vi "Settings Dialog.vi"(8 "error in (no error)":errorcluster, 11 "Settings in":T1) -> (0 "error out":errorcluster, 1 "Cancelled?":bool, 2 "UI Refresh Needed?":bool, 3 "Settings out":T1)   [LabVIEW 2022 SP3, in "Settings.lvlib"]
doc: "Dialog for selecting user specified settings."
uses:
  Settings.lvlib
  Settings.ctl
  Acquisition/Network Configuration.ctl
  Logging/Logging Configuration.ctl
  <vilib>/Utility/xml.llb/Write to XML File(string).vi
  Acquisition/Acquisition.lvlib
  Logging/Logging.lvlib
panel:
  in  "IP Address":string="127.0.0.1"
  in  "Port":dbl=5005.0
  in  "Log File Path":path
  in  "Cancel Button":bool
  in  "OK Button":bool
  # "Non visible portion of dialog (needed for connector pane)."
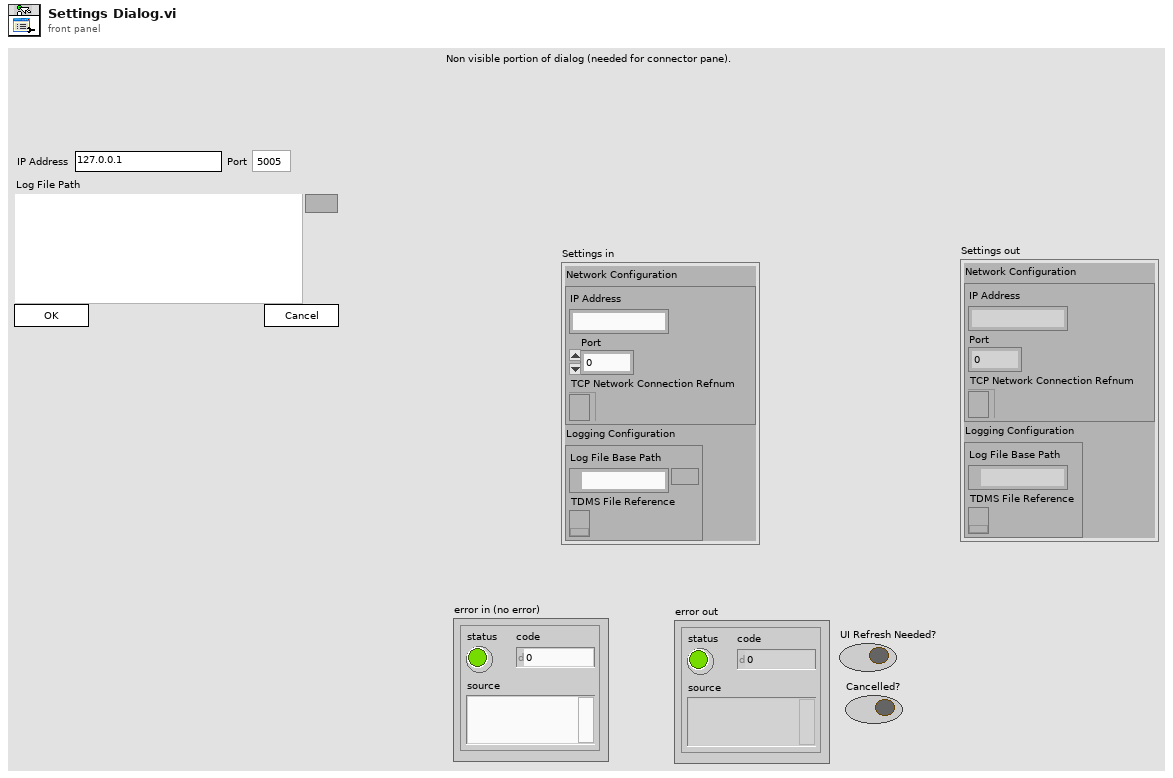
[diagram p1: front panel]
types:
  T1 = typedef "Settings.lvlib/Settings.ctl" = cluster{"Network Configuration":T2, "Logging Configuration":T3}
  T2 = typedef "Acquisition.lvlib/Network Configuration.ctl" = cluster{"IP Address":string, "Port":dbl, "TCP Network Connection Refnum":refnum<k5>}
  T3 = typedef "Logging.lvlib/Logging Configuration.ctl" = cluster{"Log File Base Path":path, "TDMS File Reference":refnum<k34>}
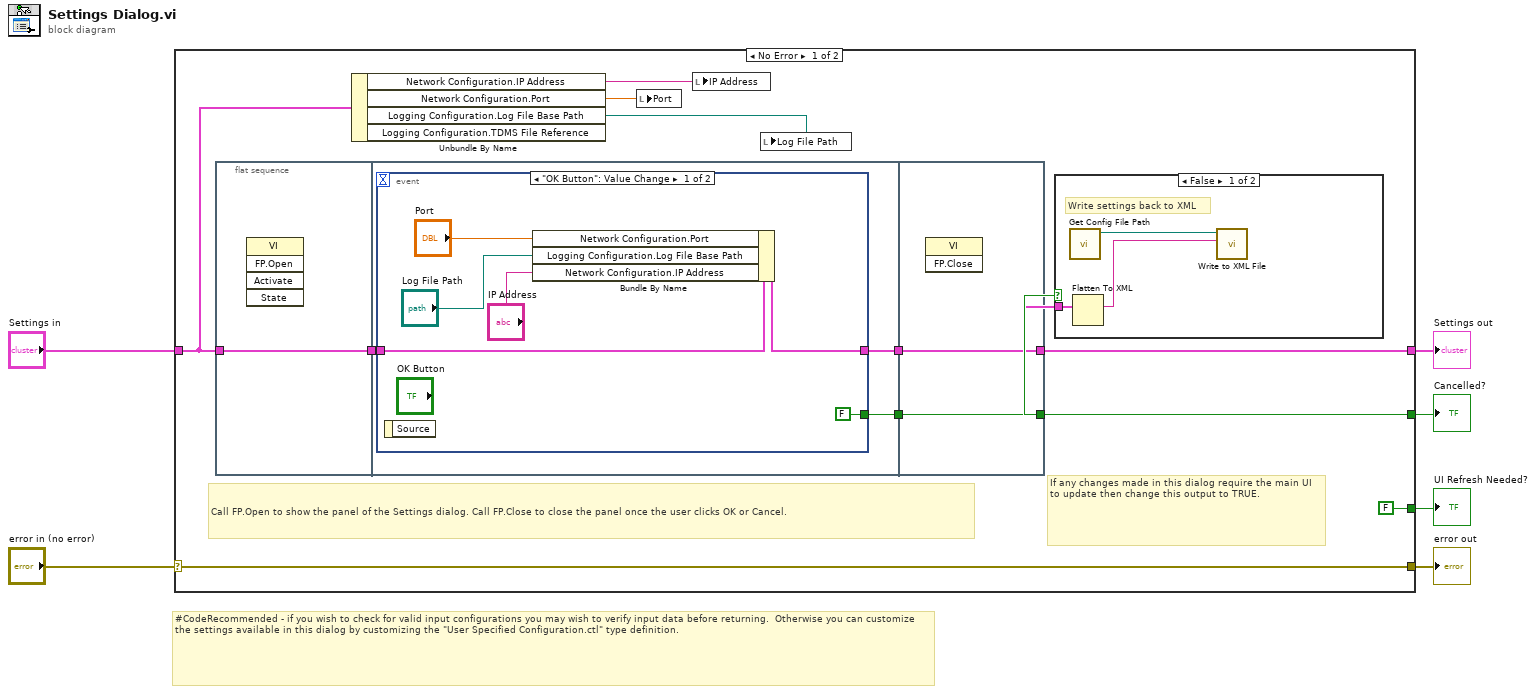
[diagram p0: block diagram]
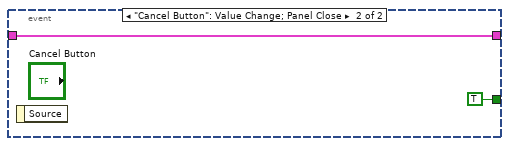
[diagram p2: hidden frame]
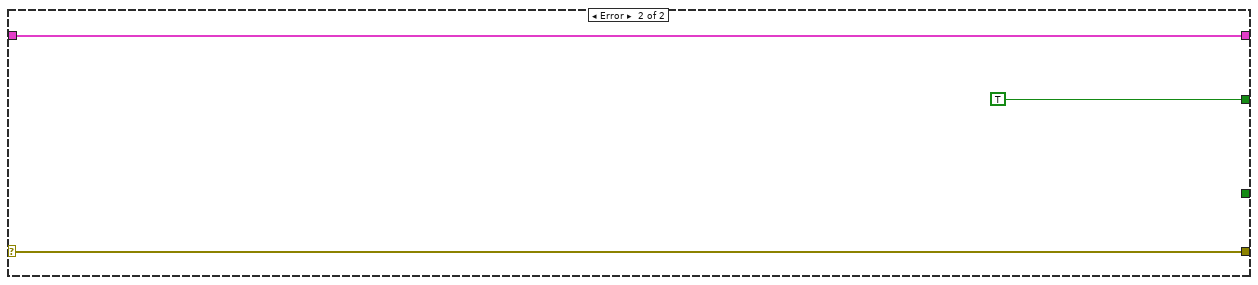
[diagram p4: hidden frame]
diagram:
  # "#CodeRecommended - if you wish to check for valid input configurations you may wish to verify input data before returning.  Otherwise you can customize the settings available in this dialog by customizing the \"User Specified Configuration.ctl\" type definition."
  n1 = case shown="No Error" "error in (no error)" {
    selector: "error in (no error)" -> [w17 w37]
    tunnel: [w17 w37] -> w5
    tunnel: "Settings in" -> [w13 w36]
    tunnel: [w14 w36] -> w3
    tunnel: [FALSE ("UI Refresh Needed?") _] -> w2
    tunnel: [w15 TRUE ("UI Refresh Needed?")] -> w1
    frame No Error {
      # "Call FP.Open to show the panel of the Settings dialog. Call FP.Close to close the panel once the user clicks OK or Cancel."
      # "If any changes made in this dialog require the main UI to update then change this output to TRUE."
      n2 = flat-sequence {
        tunnel: w13 -> [w18]
        tunnel: [w18] -> w10
        tunnel: w10 -> [w19]
        tunnel: [w21] -> w9
        tunnel: [w20] -> w8
        tunnel: [w30] -> w14
        tunnel: [w31] -> w15
        tunnel: w9 -> [w31]
        tunnel: w8 -> [w30]
        frame #0 {
          n3 = invoke class="VI" method="FP.Open"() -> ()  [unwired: 5 in, 5 out]
        }
        frame #1 {
          n4 = event shown="[0] \"OK Button\": Value Change" {
            selector: _ -> [_ _]
            dyn-events: _ -> [_ _]
            timeout: _ -> [_ _]
            tunnel: [w25 w29] -> w20
            tunnel: w19 -> [w26 w29]
            tunnel: [FALSE ("UI Refresh Needed?") TRUE ("UI Refresh Needed?")] -> w21
            event "OK Button": Value Change {
              n5 = event-data() -> ()  [unwired: 1 in, 1 out]
              n6 = Bundle By Name(cluster=w26, "Network Configuration.Port"="Port", "Logging Configuration.Log File Base Path"="Log File Path", "Network Configuration.IP Address"="IP Address") -> (w25:T1)
            }
            event "Cancel Button": Value Change; Panel Close {
              n7 = event-data() -> ()  [unwired: 1 in, 1 out]
            }
          }
        }
        frame #2 {
          n8 = invoke class="VI" method="FP.Close"() -> ()  [unwired: 3 in, 3 out]
        }
      }
      n9 = Unbundle By Name(w13) -> ("Network Configuration.IP Address"=w7:string, "Network Configuration.Port"=w12:dbl, "Logging Configuration.Log File Base Path"=w11:path)  [unwired: 1 out]
      n10 = local write "Port"(w12) -> ()
      n11 = local write "IP Address"(w7) -> ()
      n12 = local write "Log File Path"(w11) -> ()
      n13 = case shown="False" w15 {
        tunnel: w14 -> [w33 _]
        frame False {
          # "Write settings back to XML"
          n14 = call "Get Config File Path.vi"() -> ("XML File Path"=w34:path)  [unwired: 10 in, 1 out]
          n15 = Flatten To XML(6:w33) -> (2:w32:string)
          n16 = call-poly <vilib>:"Write to XML File.vi"("XML Input"=w32, "XML File Path"=w34) -> ()  [unwired: 7 in, 3 out]
        }
        frame True {
        }
      }
    }
    frame Error {
    }
  }
  "UI Refresh Needed?" <- w2
  "error out" <- w5
  "Settings out" <- w3
  "Cancelled?" <- w1
